vi "Node - Read U8 Array from Byte Buffer.vi"(8 "error in (no error)":errorcluster, 11 "Node Data In":T1) -> (0 "error out":errorcluster, 2 "U8 Array Out":u8[](array[numeric]), 3 "Node Data Out":T1)   [LabVIEW 2016, in "PXImc Router.lvlib"]
uses:
  PXImc Router.lvlib
  Controls/Node Data.ctl
  Controls/Node/Node - PXImc Parameters.ctl
  Controls/Node/Node - Writer Data.ctl
  Controls/Node/Node Ch Properties.ctl
  Controls/Data Type.ctl
  Controls/Node/Node - Readers Data.ctl
  Controls/Node/Node - Reader Data.ctl
  <vilib>/NI Veristand/VeriStand Data/Byte Buffer/Byte Buffer.lvclass
  <vilib>/NI Veristand/VeriStand Data/Byte Buffer/Byte Buffer.lvclass/Byte Buffer.ctl
  <vilib>/NI Veristand/VeriStand Data/Pointer Operations/Pointer.Read (I32).vi
  <vilib>/NI Veristand/VeriStand Data/Pointer Operations/Pointer.Read (1D U8).vi
  <vilib>/NI Veristand/VeriStand Data/Pointer Operations/Pointer.In-Place Read (I32).vi
  <vilib>/NI Veristand/VeriStand Data/Pointer Operations/Pointer.In-Place Read (1D U8).vi
  <vilib>/NI Veristand/VeriStand Data/VeriStand Data.lvlib
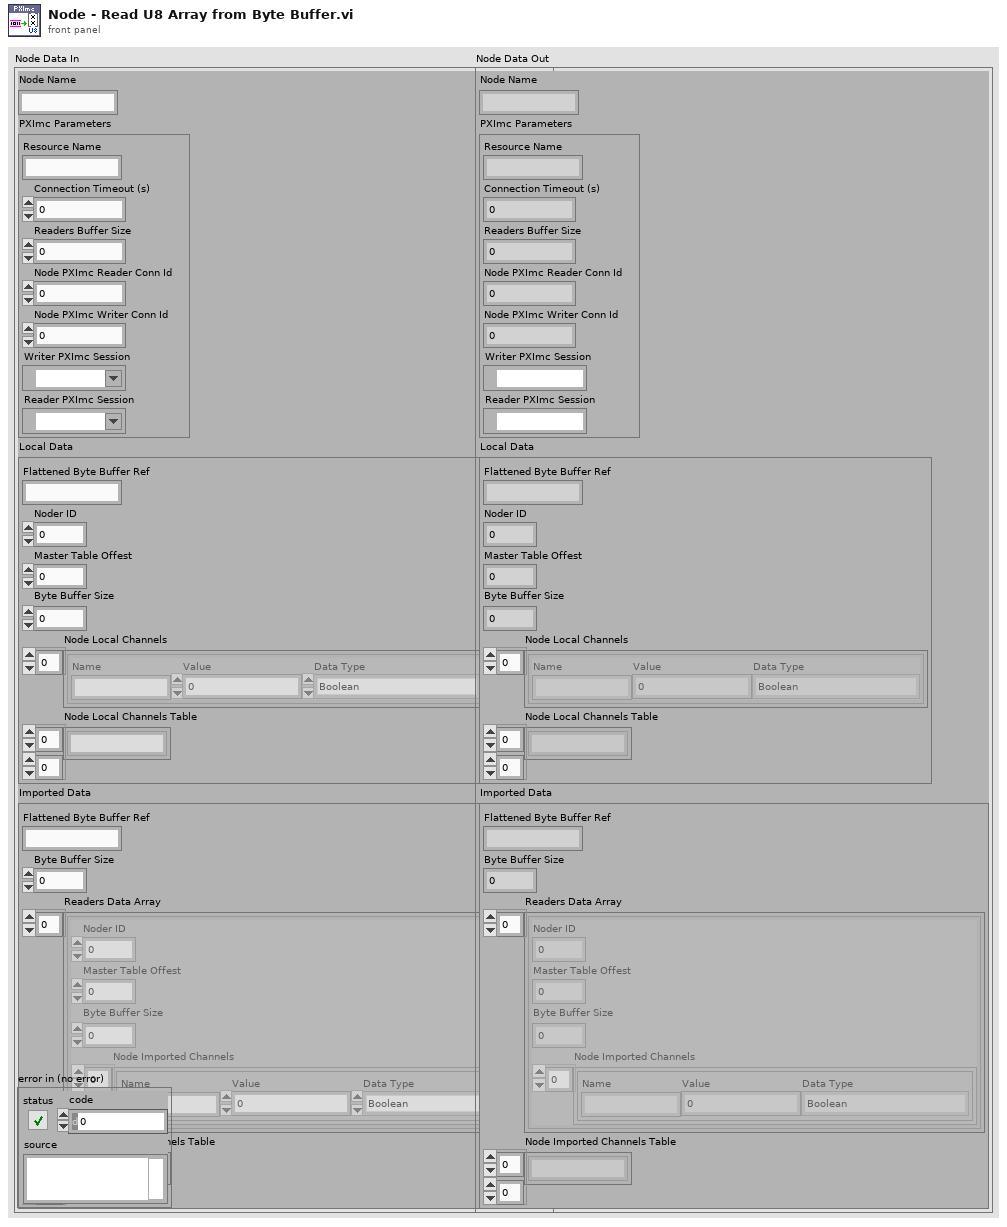
[diagram p1: front panel]
types:
  T1 = typedef "PXImc Router.lvlib/Node Data.ctl" = cluster{"Node Name":string, "PXImc Parameters":T2, "Local Data":T3, "Imported Data":T6}
  T2 = typedef "PXImc Router.lvlib/Node - PXImc Parameters.ctl" = cluster{"Resource Name":string, "Connection Timeout (s)":dbl, "Readers Buffer Size":u64, "Node PXImc Reader Conn Id":u16, "Node PXImc Writer Conn Id":u16, "Writer PXImc Session":refnum<k21>, "Reader PXImc Session":refnum<k21>}
  T3 = typedef "PXImc Router.lvlib/Node - Writer Data.ctl" = cluster{"Flattened Byte Buffer Ref":string, "Noder ID":u32, "Master Table Offest":u32, "Byte Buffer Size":u32, "Node Local Channels":T4[], "Node Local Channels Table":string[][]}
  T4 = typedef "PXImc Router.lvlib/Node Ch Properties.ctl" = cluster{"Name":string, "Value":dbl, "Data Type":T5}
  T5 = typedef "PXImc Router.lvlib/Data Type.ctl" = enum16{"Boolean", "SGL", "DBL", "I8", "I16", "I32", "I64", "U8", "U16", "U32", "U64"}
  T6 = typedef "PXImc Router.lvlib/Node - Readers Data.ctl" = cluster{"Flattened Byte Buffer Ref":string, "Byte Buffer Size":u64, "Readers Data Array":T7[], "Node Imported Channels Table":string[][]}
  T7 = typedef "PXImc Router.lvlib/Node - Reader Data.ctl" = cluster{"Noder ID":u32, "Master Table Offest":u32, "Byte Buffer Size":u64, "Node Imported Channels":T4[]}
  T8 = typedef "VeriStand Data.lvlib/Byte Buffer.lvclass/Byte Buffer.Pointers.ctl" = cluster{"buffer data ptr":u64, "buffer size ptr":u64, "byte order ptr":u64}
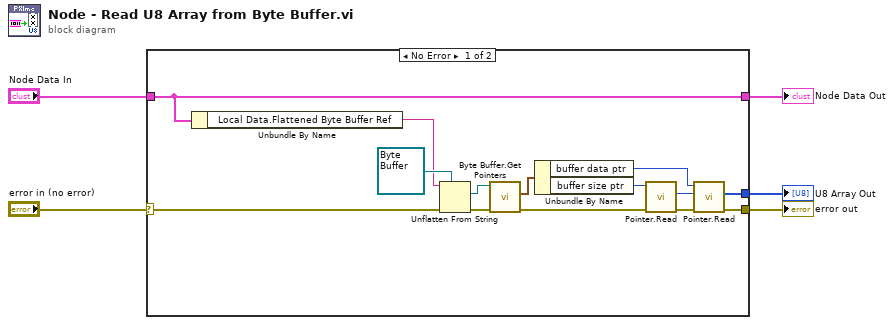
[diagram p0: block diagram]
diagram:
  n1 = case shown="No Error" "error in (no error)" {
    selector: "error in (no error)" -> [w7 w20]
    tunnel: [w19 _] -> w5
    tunnel: [w17 w20] -> w4
    tunnel: "Node Data In" -> [w11 w21]
    tunnel: [w11 w21] -> w2
    frame No Error {
      n2 = Unbundle By Name(w11) -> ("Local Data.Flattened Byte Buffer Ref"=w9:string)
      n3 = Unflatten From String(type=refnum<class "Byte Buffer.lvclass"> refnum ("Byte Buffer out"), binary string=w9, error in (no error)=w7) -> (value=w8:refnum<class "Byte Buffer.lvclass">, error out=w6:errorcluster)  [unwired: 2 in, 1 out]
      n4 = call <vilib>:"Byte Buffer.Get Pointers.vi"("error in (no error)"=w6, "Byte Buffer in"=w8) -> ("error out"=w18:errorcluster, "Byte Buffer pointers"=w16:T8)  [unwired: 7 in, 1 out]
      n5 = Unbundle By Name(w16) -> ("buffer data ptr"=w12:u64, "buffer size ptr"=w13:u64)
      n6 = call-poly <vilib>:"Pointer.Read.vi"("error in (no error)"=w18, "pointer in"=w13) -> ("error out"=w15:errorcluster, "value"=w14:i32)  [unwired: 7 in, 1 out]
      n7 = call-poly <vilib>:"Pointer.Read.vi"("error in (no error)"=w15, "count"=w14, "pointer in"=w12) -> ("error out"=w17:errorcluster, "values"=w19:u8[])  [unwired: 6 in, 1 out]
    }
    frame Error {
    }
  }
  "U8 Array Out" <- w5
  "error out" <- w4
  "Node Data Out" <- w2
